vi "Replase ALR_ON_OFF amc.vi"(8 "error in":errorcluster, 9 "message":T1, 10 "ALR_Names":string[](array[string]), 11 "ALR_ON_OFF in":refnum<data-value>) -> (0 "error out":errorcluster, 3 "ALR_ON_OFF out":refnum<data-value>)   [LabVIEW 2019, in "Alarms.lvlib"]
uses:
  Alarms.lvlib
  Ctl/ALR_ON_OFF.ctl
  <vilib>/NI/AMC/Message.ctl
  <vilib>/NI/Tools/Keyed Array/KeyedArray.ctl
  Ctl/ALR_Control.ctl
  <vilib>/NI/Tools/Keyed Array/Tools_KeyedArray.lvlib
  <vilib>/NI/AMC/AMC.lvlib
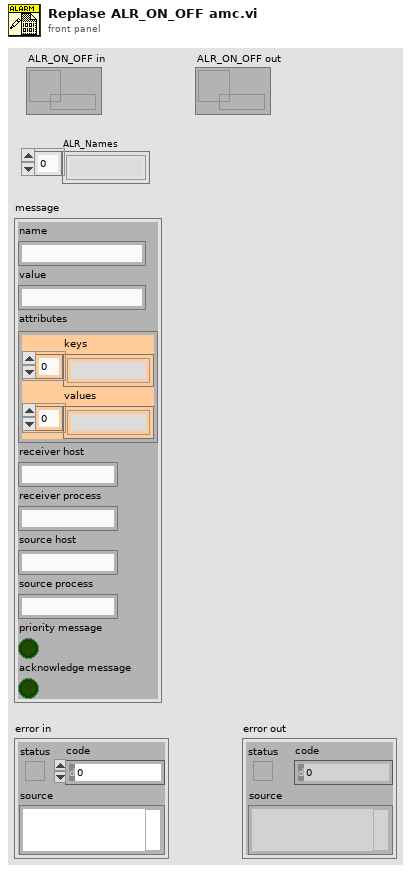
[diagram p1: front panel]
types:
  T1 = typedef "AMC.lvlib/Message.ctl" = cluster{"name":string, "value":string, "attributes":T2, "receiver host":string, "receiver process":string, "source host":string, "source process":string, "priority message":bool, "acknowledge message":bool}
  T2 = typedef "Tools_KeyedArray.lvlib/KeyedArray.ctl" = cluster{"keys":string[], "values":string[]}
  T3 = typedef "Alarms.lvlib/ALR_Control.ctl" = enum16{"UNDEFINED", "ALR_ON", "ALR_OFF", "ALR_reset", "ALR_check_ON", "ALR_reset_OFF", "ALR_check_OFF", "ALR_block_ON", "ALR_block_OFF", "ALR_Ack", "ALR_Ack_OFF"}
  T4 = typedef "Alarms.lvlib/ALR_ON_OFF.ctl" = cluster{"ALR_ON":bool[], "ALR_OFF":bool[], "ALR_reset":bool[], "ALR_check":bool[], "ALR_block":bool[], "ALR_Ack":bool[]}
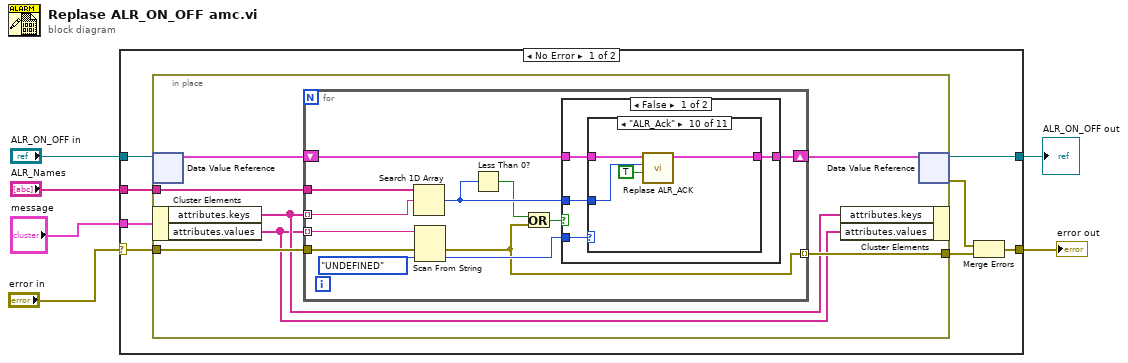
[diagram p0: block diagram]
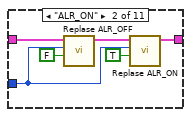
[diagram p3: hidden frame]
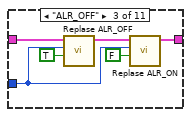
[diagram p4: hidden frame]
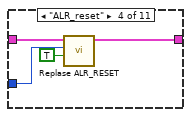
[diagram p5: hidden frame]
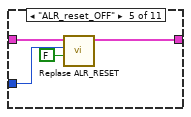
[diagram p6: hidden frame]
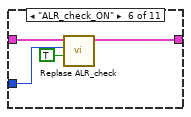
[diagram p7: hidden frame]
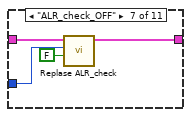
[diagram p8: hidden frame]
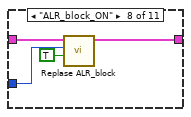
[diagram p9: hidden frame]
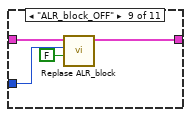
[diagram p10: hidden frame]
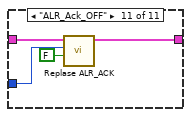
[diagram p11: hidden frame]
diagram:
  n1 = case shown="No Error" "error in" {
    selector: "error in" -> [w10 w84]
    tunnel: "ALR_ON_OFF in" -> [w14 w85]
    tunnel: [w13 w85] -> w5
    tunnel: "ALR_Names" -> [w12 _]
    tunnel: "message" -> [w11 _]
    tunnel: [w7 w84] -> w1
    frame No Error {
      n2 = in-place {
        in-place-border: w12 -> [w19]
        in-place-border: w10 -> [w18]
        in-place-border: [w17] -> w8
        n3 = in-place-dvr #1(w14) -> (w21:T4)  [unwired: 1 out]
        n4 = in-place-cluster #2(w11) -> ("attributes.keys"=w16:string[], "attributes.values"=w15:string[])
        n5 = for {
          shift-right: [w32] -> w20
          shift-left: w21 -> [w33]
          tunnel: w15 -> [w30] mode=indexing
          tunnel: w16 -> [w28] mode=indexing
          tunnel: w19 -> [w27]
          tunnel: w18 -> [w23]
          tunnel: [w22] -> w17 mode=indexing
          n6 = Search 1D Array(1D array=w27, element=w28) -> (index of element=w26:i32)  [unwired: 1 in]
          n7 = Scan From String(input string=w30, error in=w23, default 1=ALR_Control."UNDEFINED" ("ALR_Control")) -> (error out=w22:errorcluster, output 1=w29:T3)  [unwired: 2 in, 2 out]
          n8 = Less Than 0?(x=w26) -> (x < 0?=w24:bool)
          n9 = Or(x=w24, y=w22) -> (x .or. y?=w25:bool)
          n10 = case shown="False" w25 {
            tunnel: w33 -> [w37 w83]
            tunnel: [w36 w83] -> w32
            tunnel: w29 -> [w35 _]
            tunnel: w26 -> [w34 _]
            frame False {
              n11 = case shown="\"ALR_Ack\"" w35 {
                tunnel: w37 -> [w38 w41 w47 w54 w58 w62 w66 w70 w74 w78 w82]
                tunnel: [w38 w44 w50 w53 w57 w61 w65 w69 w73 w77 w81] -> w36
                tunnel: w34 -> [_ w40 w46 w51 w55 w59 w63 w67 w71 w75 w79]
                frame "UNDEFINED", Default {
                }
                frame "ALR_ON" {
                  n12 = call "Replase ALR_OFF.vi"("ALR_OFF"=FALSE ("ALR_ON"), "N"=w40, "ALR_ON_OFF in"=w41) -> ("ALR_ON_OFF out"=w39:T4)  [unwired: 8 in]
                  n13 = call "Replase ALR_ON.vi"("ALR_ON"=TRUE, "N"=w40, "ALR_ON_OFF in"=w39) -> ("ALR_ON_OFF out"=w44:T4)  [unwired: 8 in]
                }
                frame "ALR_OFF" {
                  n14 = call "Replase ALR_OFF.vi"("ALR_OFF"=TRUE ("ALR_ON"), "N"=w46, "ALR_ON_OFF in"=w47) -> ("ALR_ON_OFF out"=w45:T4)  [unwired: 8 in]
                  n15 = call "Replase ALR_ON.vi"("ALR_ON"=FALSE, "N"=w46, "ALR_ON_OFF in"=w45) -> ("ALR_ON_OFF out"=w50:T4)  [unwired: 8 in]
                }
                frame "ALR_reset" {
                  n16 = call "Replase ALR_RESET.vi"("ALR_RST"=TRUE, "N"=w51, "ALR_ON_OFF in"=w54) -> ("ALR_ON_OFF out"=w53:T4)  [unwired: 8 in]
                }
                frame "ALR_reset_OFF" {
                  n17 = call "Replase ALR_RESET.vi"("ALR_RST"=FALSE, "N"=w55, "ALR_ON_OFF in"=w58) -> ("ALR_ON_OFF out"=w57:T4)  [unwired: 8 in]
                }
                frame "ALR_check_ON" {
                  n18 = call "Replase ALR_check.vi"("ALR_check"=TRUE, "N"=w59, "ALR_ON_OFF in"=w62) -> ("ALR_ON_OFF out"=w61:T4)  [unwired: 8 in]
                }
                frame "ALR_check_OFF" {
                  n19 = call "Replase ALR_check.vi"("ALR_check"=FALSE, "N"=w63, "ALR_ON_OFF in"=w66) -> ("ALR_ON_OFF out"=w65:T4)  [unwired: 8 in]
                }
                frame "ALR_block_ON" {
                  n20 = call "Replase ALR_block.vi"("ALR_block"=TRUE, "N"=w67, "ALR_ON_OFF in"=w70) -> ("ALR_ON_OFF out"=w69:T4)  [unwired: 8 in]
                }
                frame "ALR_block_OFF" {
                  n21 = call "Replase ALR_block.vi"("ALR_block"=FALSE ("ALR_check"), "N"=w71, "ALR_ON_OFF in"=w74) -> ("ALR_ON_OFF out"=w73:T4)  [unwired: 8 in]
                }
                frame "ALR_Ack" {
                  n22 = call "Replase ALR_ACK.vi"("ALR_ACK"=TRUE, "N"=w75, "ALR_ON_OFF in"=w78) -> ("ALR_ON_OFF out"=w77:T4)  [unwired: 8 in]
                }
                frame "ALR_Ack_OFF" {
                  n23 = call "Replase ALR_ACK.vi"("ALR_ACK"=FALSE, "N"=w79, "ALR_ON_OFF in"=w82) -> ("ALR_ON_OFF out"=w81:T4)  [unwired: 8 in]
                }
              }
            }
            frame True {
            }
          }
        }
        n24 = in-place-cluster #2("attributes.keys"=w16, "attributes.values"=w15) -> ()  [unwired: 1 out]
        n25 = in-place-dvr #1(w20) -> (w13:refnum<data-value>, w9:errorcluster)
      }
      n26 = Merge Errors(w9, w8) -> (w7:errorcluster)
    }
    frame Error {
    }
  }
  "ALR_ON_OFF out" <- w5
  "error out" <- w1
